vi "Get Nodes in Path.vi"(8 "error in (no error)":errorcluster, 10 "path references":refnum<data-value>[](array[refnum]), 11 "map reference in":refnum<data-value>) -> (0 "error out":errorcluster, 2 "nodes":cluster{"name":string, "coordinates":dbl[]}[](array[cluster]), 3 "map reference out":refnum<data-value>)   [LabVIEW 2017, in "NI_Robotics_DirectedGraphWorldMap.lvclass"]
doc: "Returns the names and coordinates of the <B>nodes</B> along a path through a directed graph map."
uses:
  <vilib>/robotics/Navigation/shared/WorldMap/DirectedGraphWorldMap/NI_Robotics_DirectedGraphWorldMap.lvclass
  <vilib>/robotics/Navigation/shared/MapNode/AbstractAstarNode/NI_Robotics_AbstractAstarNode.lvclass
  <vilib>/robotics/Navigation/shared/MapNode/DirectedGraphMapNode/NI_Robotics_DirectedGraphMapNode.lvclass
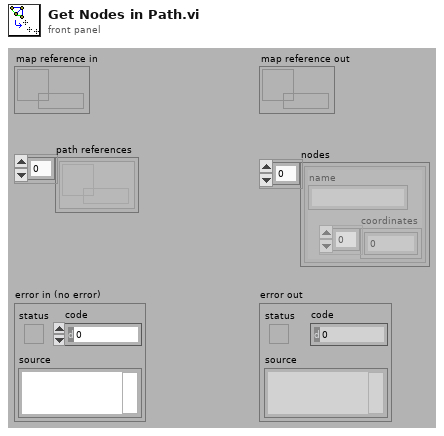
[diagram p1: front panel]
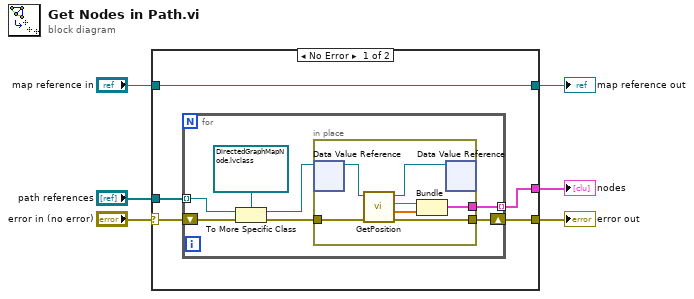
[diagram p0: block diagram]
diagram:
  n1 = case shown="No Error" "error in (no error)" {
    selector: "error in (no error)" -> [w10 w26]
    tunnel: "path references" -> [w11 _]
    tunnel: [w9 w27] -> w5
    tunnel: "map reference in" -> [w9 w27]
    tunnel: [w8 w26] -> w2
    tunnel: [w7 _] -> w1
    frame No Error {
      n2 = for {
        tunnel: w11 -> [w17] mode=indexing
        shift-right: [w14] -> w8
        shift-left: w10 -> [w18]
        tunnel: [w12] -> w7 mode=indexing
        n3 = To More Specific Class(target class=refnum<data-value> refnum ("Node ref"), reference=w17, error in=w18) -> (specific class reference=w16:refnum<data-value>, error out=w15:errorcluster)
        n4 = in-place {
          in-place-border: w15 -> [w23]
          in-place-border: [w22] -> w14
          in-place-border: [w19] -> w12
          n5 = in-place-dvr #1(w16) -> (w25:refnum<class "NI_Robotics_DirectedGraphMapNode.lvclass">)  [unwired: 1 out]
          n6 = call <vilib>:"GetPosition.vi"("error in (no error)"=w23, "DirectedGraphMapNode in"=w25) -> ("error out"=w22:errorcluster, "coordinates"=w21:dbl[], "name"=w20:string, "DirectedGraphMapNode out"=w24:refnum<class "NI_Robotics_DirectedGraphMapNode.lvclass">)  [unwired: 6 in]
          n7 = Bundle("name"=w20, "coordinates"=w21) -> (w19:cluster{"name":string, "coordinates":dbl[]})  [unwired: 1 in]
          n8 = in-place-dvr #1(w24) -> ()  [unwired: 2 out]
        }
      }
    }
    frame Error {
    }
  }
  "map reference out" <- w5
  "error out" <- w2
  "nodes" <- w1
